vi "Status display interface.vi"(8 "error in (no error)":errorcluster, 11 "Message":string) -> (0 "error out":errorcluster)   [LabVIEW 2013]
uses:
  Global Variables/gl_Queues.vi
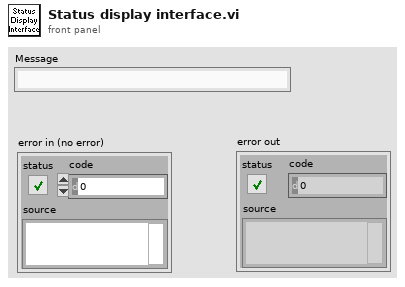
[diagram p1: front panel]
types:
  T1 = typedef "All Message Queues.ctl" = cluster{"UI queue":refnum<queue>, "Acq. queue":refnum<queue>, "Logging queue":refnum<queue>}
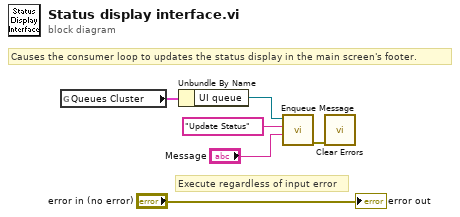
[diagram p0: block diagram]
diagram:
  # "Execute regardless of input error"
  # "Causes the consumer loop to updates the status display in the main screen's footer."
  n1 = global read "gl_Queues.vi" "Queues Cluster"() -> (w5:T1)
  n2 = Unbundle By Name(w5) -> ("UI queue"=w6:refnum<queue>)
  n3 = call "Enqueue Message.vi"("Message Data"="Message", "Message"="Update Status", "Queue"=w6) -> ("error out"=w3:errorcluster)  [unwired: 7 in, 1 out]
  n4 = call <vilib>:"Clear Errors.vi"("error in (no error)"=w3) -> ()  [unwired: 6 in, 1 out]
  "error out" <- "error in (no error)"
